vi "Trigger_Receiver.vi"(0 "Trigger Execute Experiment":bool, 1 "Trigger digitals transfer":bool, 2 "Trigger analogues transfer":bool, 3 "Trigger Indexes Write":bool, 4 "Trigger Write Digitals":bool, 5 "Trigger Write Analogue":bool, 6 "Trigger Take Snap":bool, 7 "Trigger flush FIFOs":bool, 9 "Trigger Repetitions update":bool, 11 "Trigger Slow Mosaic":bool, 13 "Trigger Fast Mosaic":bool) -> (26 "Action":T1(ring), 27 "Triggered":bool)   [LabVIEW 2024]
panel:
  in  "Trigger Acquisition":bool
  out "Analogues array":T2
  out "Digitals array":T3
  out "Error code":u8
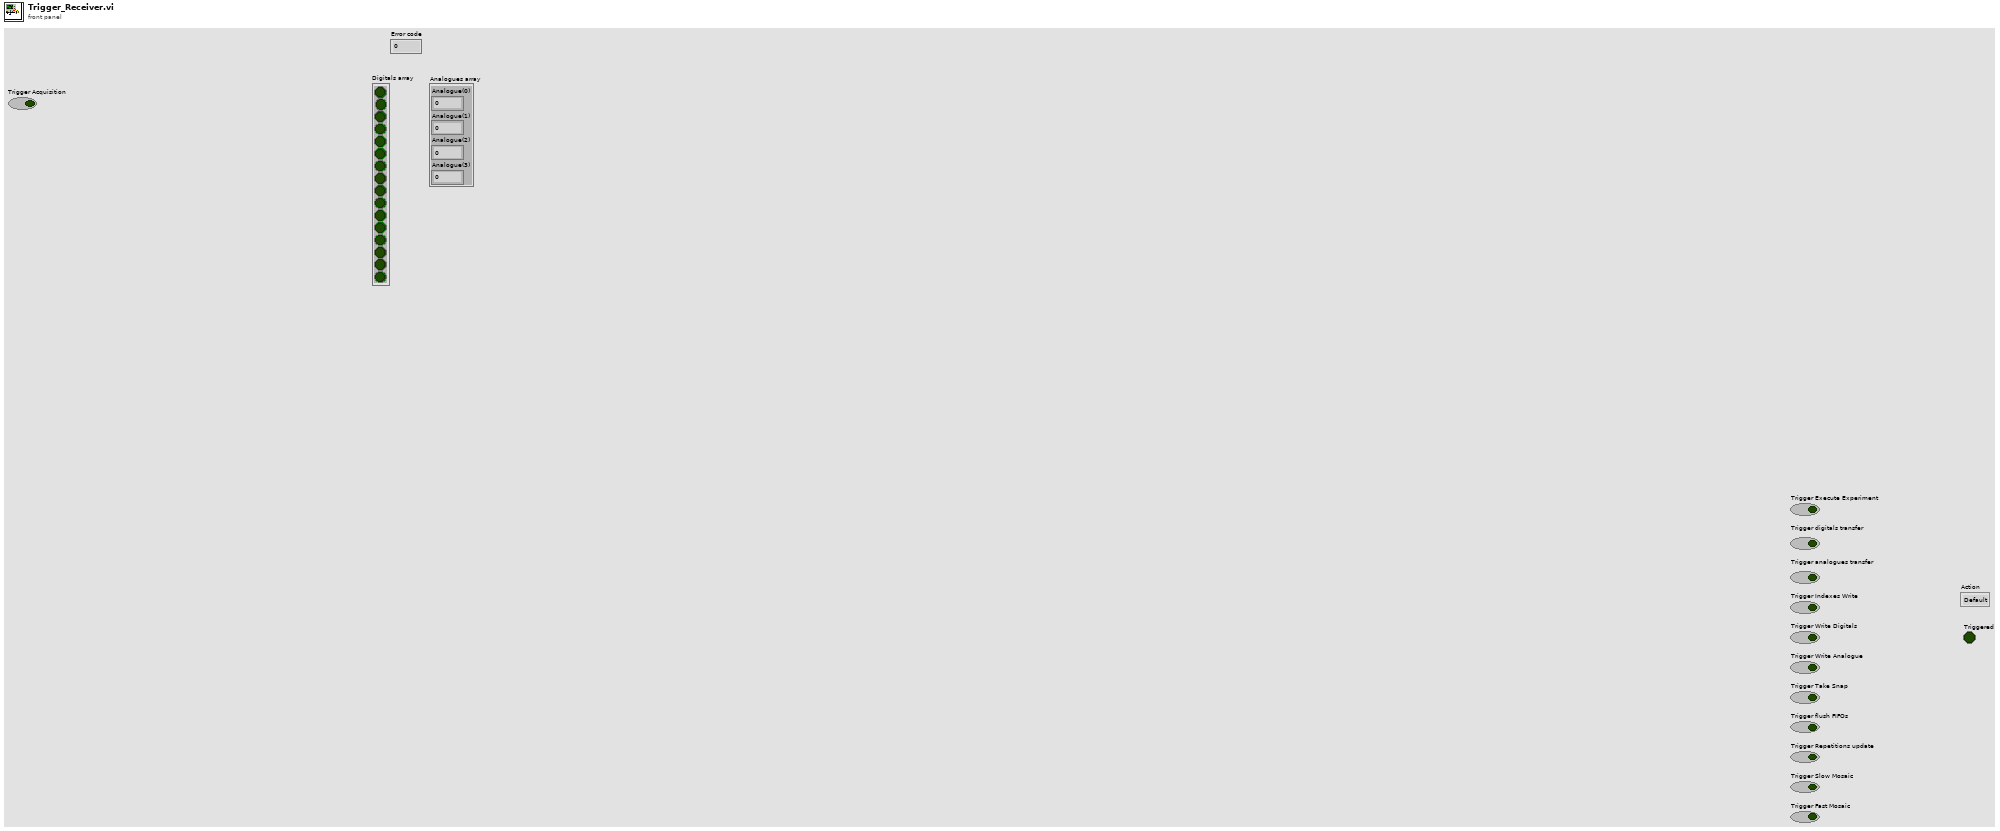
[diagram p1: front panel]
types:
  T1 = enum8{"Default", "Executing Experiment", "Transfering Digitals", "Transfering Analogues", "Writing Indexes", "Writing Digitals", "Writing Analogue", "Taking Snap", "Flushing FIFOs", "Updating Repetitions", ""}
  T2 = cluster{"Analogue(0)":i16, "Analogue(1)":i16, "Analogue(2)":i16, "Analogue(3)":i16}
  T3 = cluster{"Digital[0]":bool, "Digital[1]":bool, "Digital[2]":bool, "Digital[3]":bool, "Digital[4]":bool, "Digital[5]":bool, "Digital[6]":bool, "Digital[7]":bool, "Digital[8]":bool, "Digital[9]":bool, "Digital[10]":bool, "Digital[11]":bool, "Digital[12]":bool, "Digital[13]":bool, "Digital[14]":bool, "Digital[15]":bool}
  T4 = enum8{"Default", "Executing Experiment", "Transfering Digitals", "Transfering Analogues", "Writing Indexes", "Writing Digitals", "Writing Analogue", "Taking Snap", "Flushing FIFOs", "Updating Repetitions", "Running Slow Mosaic", "Running Fast Mosaic"}
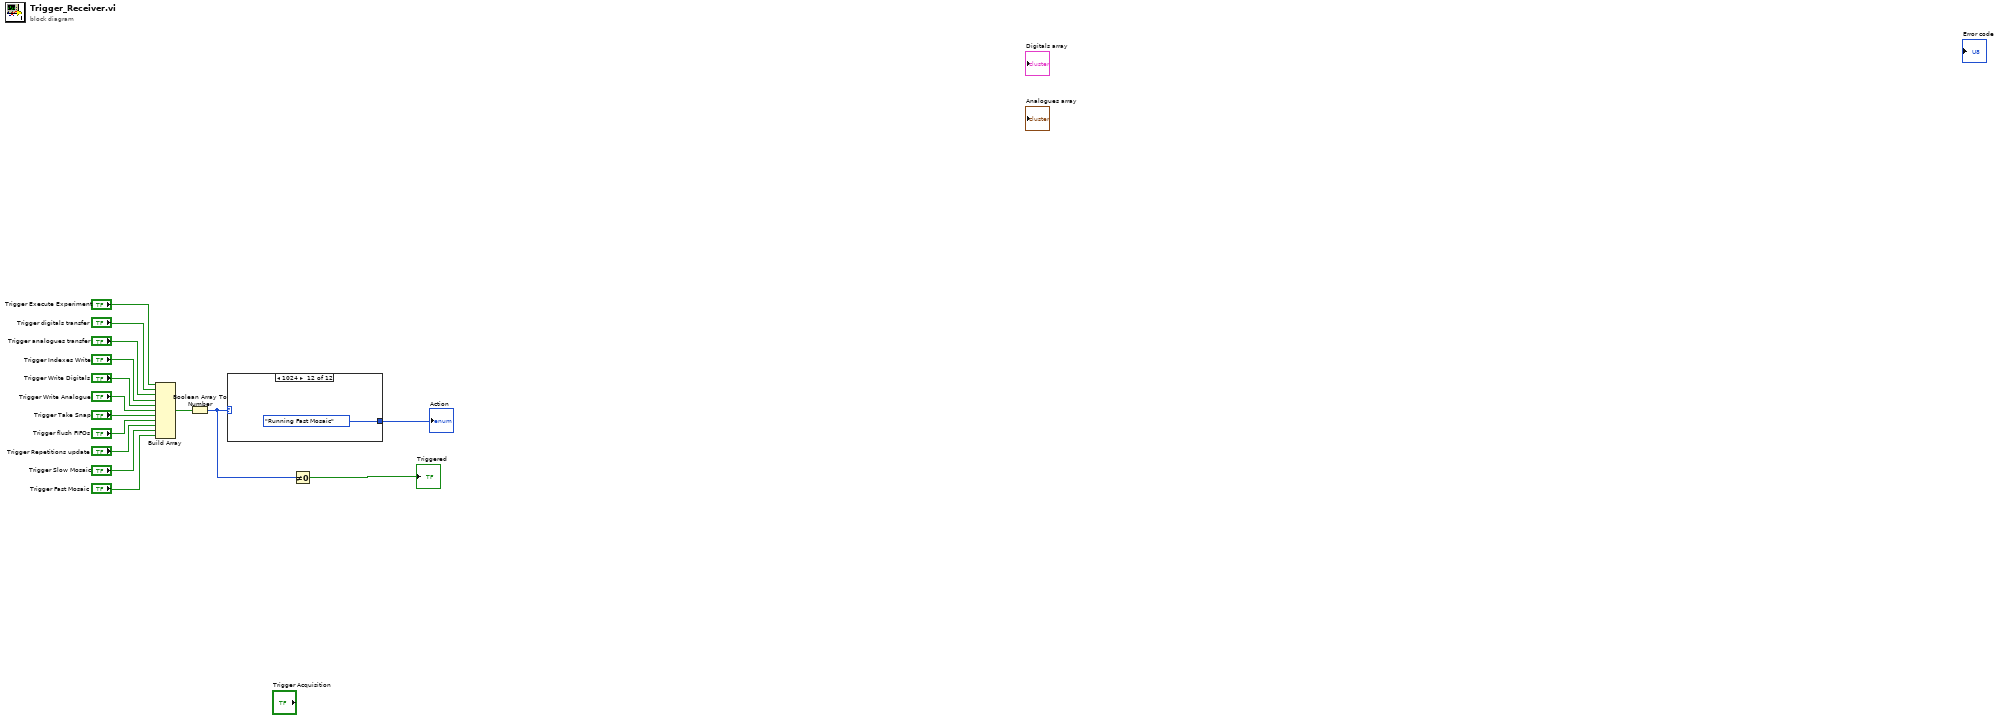
[diagram p0: block diagram]
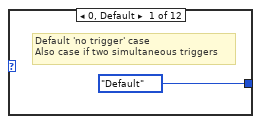
[diagram p2: hidden frame]
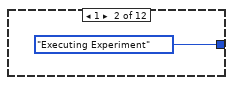
[diagram p3: hidden frame]
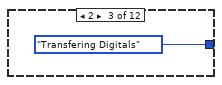
[diagram p4: hidden frame]
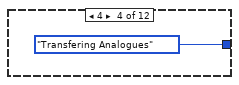
[diagram p5: hidden frame]
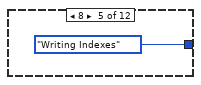
[diagram p6: hidden frame]
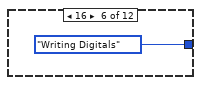
[diagram p7: hidden frame]
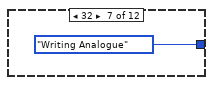
[diagram p8: hidden frame]
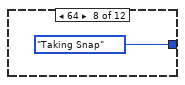
[diagram p9: hidden frame]
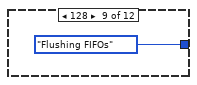
[diagram p10: hidden frame]
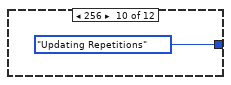
[diagram p11: hidden frame]
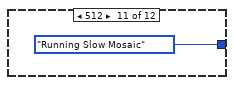
[diagram p12: hidden frame]
diagram:
  n1 = Build Array("Trigger Execute Experiment", "Trigger digitals transfer", "Trigger analogues transfer", "Trigger Indexes Write", "Trigger Write Digitals", "Trigger Write Analogue", "Trigger Take Snap", "Trigger flush FIFOs", "Trigger Repetitions update", "Trigger Slow Mosaic", "Trigger Fast Mosaic") -> (w14:bool[])
  n2 = Boolean Array To Number(Boolean array=w14) -> (number=w5:u16)
  n3 = case "Action" shown="1024" w5 {
    tunnel: [T1."Default" ("Action") T1."Executing Experiment" ("Action") T1."Transfering Digitals" ("Action") T1."Transfering Analogues" ("Action") T1."Writing Indexes" ("Action") T1."Writing Digitals" ("Action") T1."Writing Analogue" ("Action") T1."Taking Snap" ("Action") T1."Flushing FIFOs" ("Action") T4."Updating Repetitions" ("Action") T4."Running Slow Mosaic" ("Action") T4."Running Fast Mosaic" ("Action")] -> w3
    frame 0, Default {
      # "Default 'no trigger' case \nAlso case if two simultaneous triggers"
    }
    frame 1 {
    }
    frame 2 {
    }
    frame 4 {
    }
    frame 8 {
    }
    frame 16 {
    }
    frame 32 {
    }
    frame 64 {
    }
    frame 128 {
    }
    frame 256 {
    }
    frame 512 {
    }
    frame 1024 {
    }
  }
  "Action" <- w3
  n4 = Not Equal To 0?(x=w5) -> (x != 0?=→"Triggered":bool)
